vi "ITX to TDMS.vi"(8 "error in (no error)":errorcluster, 9 "Single File? [T]":bool=TRUE, 10 "Path":path, 11 "Conversion.lvclass":refnum<class "Conversion.lvclass">) -> (0 "error out":errorcluster, 1 "Not Equal?":bool, 3 "Conversion.lvclass out":refnum<class "Conversion.lvclass">)   [LabVIEW 2016, in "Conversion.lvclass"]
uses:
  Conversion.lvclass
  Data/Typedefs/File Type--enum.ctl
  Conversion.lvclass/Conversion.ctl
  Data/Typedefs/Operation--enum.ctl
  Data/Data.lvclass
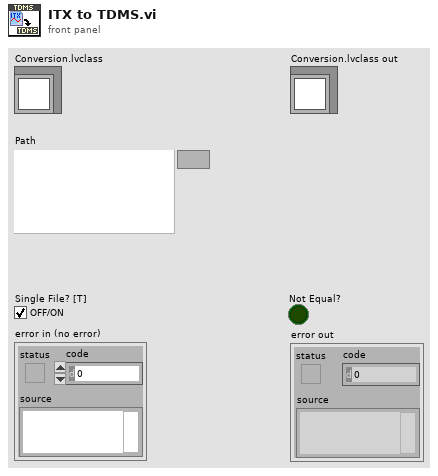
[diagram p1: front panel]
types:
  T1 = typedef "Data.lvclass/File Type--enum.ctl" = enum16{"DAT", "ITX", "HDF5", "TDMS", "VI", "PGSQL"}
  T2 = typedef "Data.lvclass/Operation--enum.ctl" = enum16{"Read", "Write", "Write + Append"}
  T3 = typedef "Data.lvclass/Dictionary--cluster.ctl" = cluster{"key":string, "value":variant}
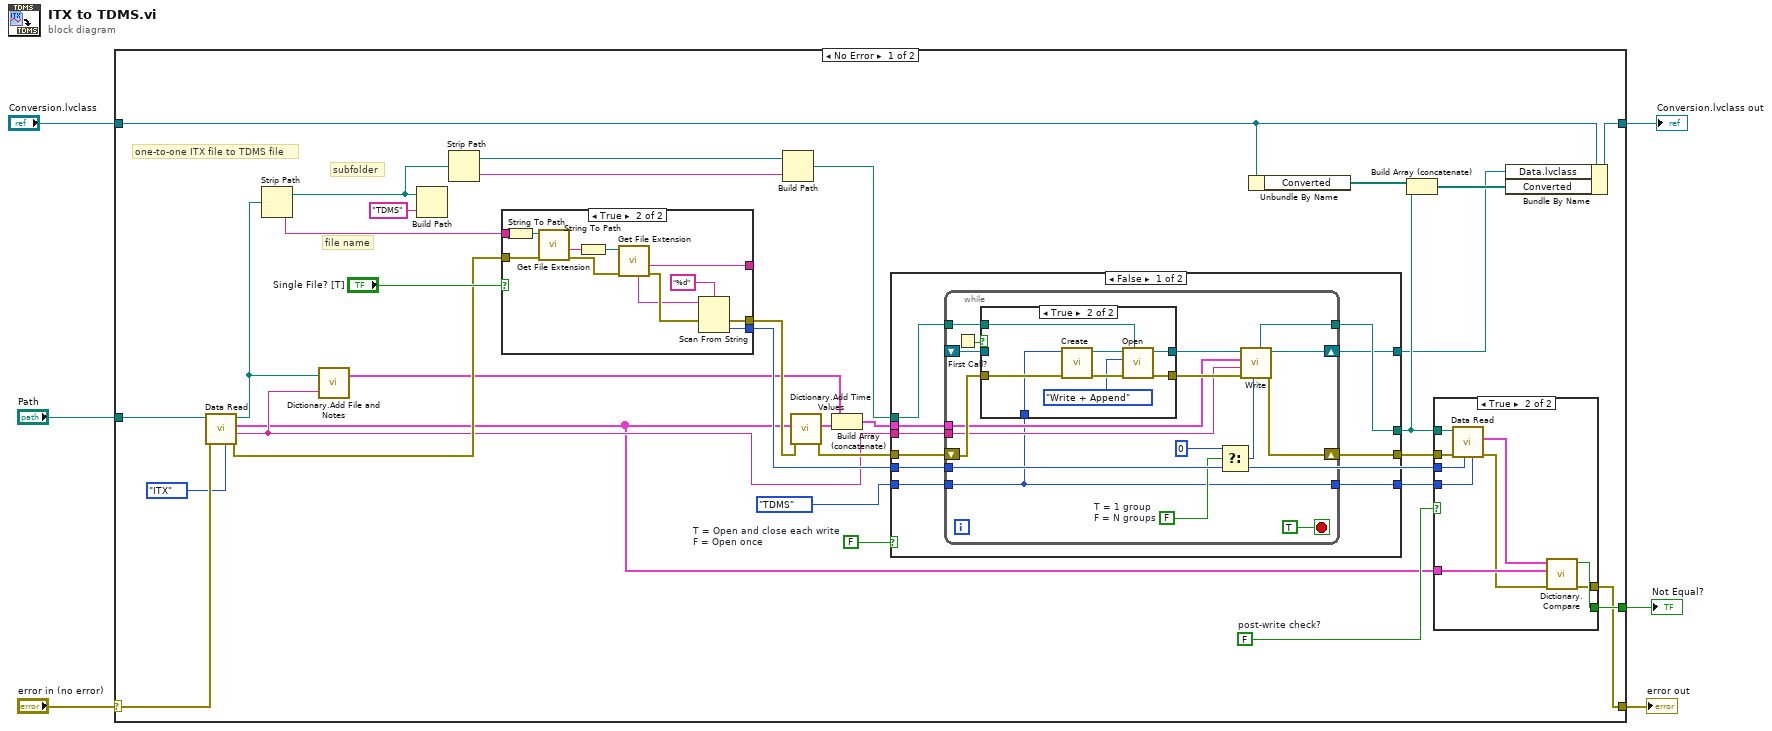
[diagram p0: block diagram]
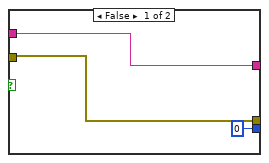
[diagram p3: hidden frame]
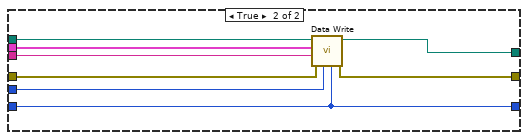
[diagram p5: hidden frame]
diagram:
  n1 = case shown="No Error" "error in (no error)" {
    selector: "error in (no error)" -> [w38 w110]
    tunnel: [w34 w110] -> w5
    tunnel: "Path" -> [w39 _]
    tunnel: [w35 _] -> w3
    tunnel: [w13 _] -> w2
    tunnel: "Conversion.lvclass" -> [w11 _]
    frame No Error {
      w18 = FALSE  # post-write check?
      w29 = FALSE  # T = Open and close each write F = Open once
      # "file name"
      # "subfolder"
      # "one-to-one ITX file to TDMS file"
      n2 = call "Data Read.vi"("File Type"=File_Type--enum."ITX", "error in (no error)"=w38, "path"=w39) -> ("error out"=w28:errorcluster, "Notes"=w23:string, "Data (Dictionary)"=w12:T3[], "path out"=w24:path)  [unwired: 5 in]
      n3 = Strip Path(path=w24) -> (stripped path=w17:path, name=w15:string)
      n4 = call "Dictionary.Add File and Notes.vi"("Notes"=w23, "Path"=w24) -> ("Dictionary"=w19:T3[])  [unwired: 1 in]
      n5 = Build Path(base path=w17, name or relative path="TDMS") -> ()  [unwired: 1 out]
      n6 = Strip Path(path=w17) -> (stripped path=w16:path, name=w14:string)
      n7 = case shown="True" "Single File? [T]" {
        tunnel: w28 -> [w50 w64]
        tunnel: w15 -> [w52 w61]
        tunnel: [w52 w53] -> _
        tunnel: [0 w54] -> w31
        tunnel: [w50 w59] -> w26
        frame False {
        }
        frame True {
          n8 = String To Path(string=w61) -> (path=w60:path)
          n9 = call <vilib>:"Get File Extension.vi"("error in (no error)"=w64, "file"=w60) -> ("error out"=w58:errorcluster, "filename without extension"=w62:string)  [unwired: 8 out]
          n10 = String To Path(string=w62) -> (path=w63:path)
          n11 = call <vilib>:"Get File Extension.vi"("error in (no error)"=w58, "file"=w63) -> ("error out"=w56:errorcluster, "filename without extension"=w53:string, "unmodified file extension"=w55:string)  [unwired: 7 out]
          n12 = Scan From String(format string="%d", input string=w55, error in=w56) -> (error out=w59:errorcluster, output 1=w54:i32)  [unwired: 2 in, 2 out]
        }
      }
      n13 = Build Path(base path=w16, name or relative path=w14) -> (appended path=w33:path)
      n14 = call "Dictionary.Add Time Values.vi"("error in (no error)"=w26, "Data (Dictionary)"=w12) -> ("error out"=w25:errorcluster, "Dictionary"=w27:T3[])  [unwired: 8 in]
      n15 = Build Array (concatenate)(w19, w27) -> (w20:T3[])
      n16 = case shown="False" w29 {
        tunnel: w23 -> [w71 w109]
        tunnel: [w67 w108] -> w8
        tunnel: [w73 w107] -> w36
        tunnel: w20 -> [w72 w106]
        tunnel: w25 -> [w74 w105]
        tunnel: w33 -> [w68 w104]
        tunnel: [w69 w102] -> w22
        tunnel: w31 -> [w70 w103]
        tunnel: [w66 _] -> w7
        tunnel: File_Type--enum."TDMS" ("File Type") -> [w65 w102]
        frame False {
          n17 = while {
            tunnel: w72 -> [w87]
            tunnel: w71 -> [w86]
            tunnel: w70 -> [w78]
            tunnel: [w75] -> w69
            tunnel: w68 -> [w85]
            shift-right: [w88] -> w73
            shift-left: w74 -> [w89]
            shift-right: [w84] -> w66
            shift-left: _ -> [w82]
            tunnel: [w80] -> w67
            tunnel: w65 -> [w75]
            stop <- TRUE stop-if-true
            w77 = FALSE  # T = 1 group F = N groups
            n18 = First Call?() -> (First Call?: T/F=w83:bool)
            n19 = case shown="True" w83 {
              tunnel: [w92 w101] -> w91
              tunnel: [w93 w100] -> w90
              tunnel: w89 -> [w92 w97]
              tunnel: w75 -> [_ w96]
              tunnel: w85 -> [_ w95]
              tunnel: w82 -> [w93 _]
              frame False {
              }
              frame True {
                n20 = call "Create.vi"("error in (no error)"=w97, "File Type"=w96) -> ("error out"=w98:errorcluster, "Data out"=w99:refnum<class "Data.lvclass">)  [unwired: 8 in]
                n21 = call-dynamic "Open.vi"("Path"=w95, "error in (no error)"=w98, "Operation"=Operation--enum."Write + Append", "Data in"=w99) -> ("error out"=w101:errorcluster, "Data out"=w100:refnum<class "Data.lvclass">)  [unwired: 6 in]
              }
            }
            n22 = Select(t=0 ("Append Index"), s=w77, f=w78) -> (s? t:f=w76:i32)
            n23 = call-dynamic "Write.vi"("Append Index"=w76, "error in (no error)"=w91, "Notes"=w86, "Data (Dictionary)"=w87, "Data in"=w90) -> ("error out"=w88:errorcluster, "Data out"=w84:refnum<class "Data.lvclass">, "Path out"=w80:path)  [unwired: 4 in]
          }
        }
        frame True {
          n24 = call "Data Write.vi"("File Type"=w102, "Append Index"=w103, "error in (no error)"=w105, "Notes"=w109, "Data (Dictionary)"=w106, "path"=w104) -> ("error out"=w107:errorcluster, "path out"=w108:path)  [unwired: 4 in]
        }
      }
      n25 = Unbundle By Name(w11) -> ("Converted"=w10:path[])
      n26 = Build Array (concatenate)(w10, w8) -> (w9:path[])
      n27 = case shown="True" w18 {
        tunnel: w8 -> [_ w49]
        tunnel: w36 -> [w40 w48]
        tunnel: [_ w47] -> w35
        tunnel: [w40 w46] -> w34
        tunnel: w31 -> [_ w45]
        tunnel: w12 -> [_ w44]
        tunnel: w22 -> [_ w43]
        frame False {
        }
        frame True {
          n28 = call "Data Read.vi"("File Type"=w43, "Append Index"=w45, "error in (no error)"=w48, "path"=w49) -> ("error out"=w42:errorcluster, "Data (Dictionary)"=w41:T3[])  [unwired: 4 in, 2 out]
          n29 = call "Dictionary.Compare.vi"("error in (no error)"=w42, "Original Data (Dictionary)"=w44, "Converted Data (Dictionary)"=w41) -> ("error out"=w46:errorcluster, "Not Equal?"=w47:bool)  [unwired: 7 in]
        }
      }
      n30 = Bundle By Name(cluster=w11, "Data.lvclass"=w7, "Converted"=w9) -> (w13:refnum<class "Conversion.lvclass">)
    }
    frame Error {
    }
  }
  "error out" <- w5
  "Not Equal?" <- w3
  "Conversion.lvclass out" <- w2
